vi "Send.vi"(7 "Motors input":refnum<vi>[](array[refnum]), 8 "Error In":errorcluster, 11 "VISA resource name":refnum<visa-resource-name>) -> (0 "Error Out":errorcluster, 3 "VISA resource name out":refnum<visa-resource-name>)   [LabVIEW 2013]
panel:
  out "return count":u32
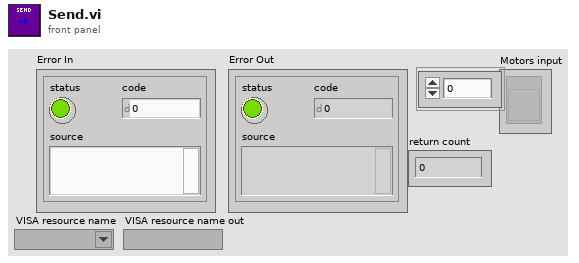
[diagram p1: front panel]
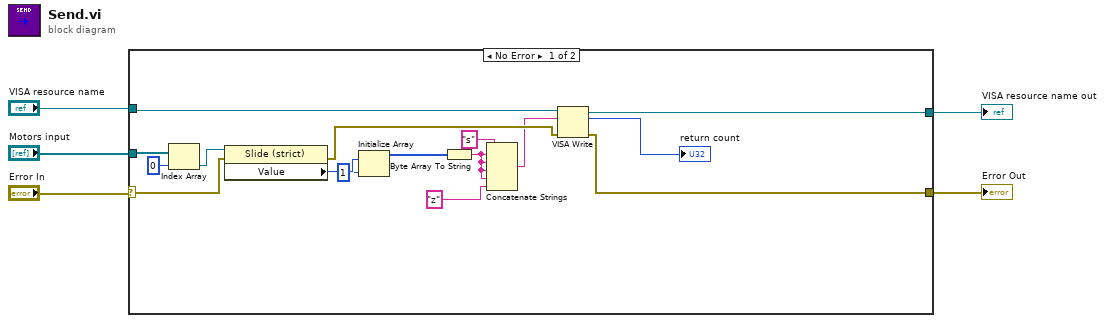
[diagram p0: block diagram]
diagram:
  n1 = case shown="No Error" "Error In" {
    selector: "Error In" -> [w15 w23]
    tunnel: [w11 w23] -> w4
    tunnel: "VISA resource name" -> [w13 w22]
    tunnel: "Motors input" -> [w21 _]
    tunnel: [w14 w22] -> w1
    frame No Error {
      n2 = Index Array(array=w21, index=0) -> (element=w19:refnum<vi>)
      n3 = property class="Slide (strict)"(reference=w19, error in=w15) -> (error out=w12:errorcluster, "Value"=w18:u8)  [unwired: 1 out]
      n4 = Initialize Array(w18, 1 ("dimension size")) -> (w16:u8[])
      n5 = Byte Array To String(unsigned byte array=w16) -> (string=w7:string)
      n6 = Concatenate Strings("s" ("string"), w7, w7, w7, w7, "z" ("string")) -> (w9:string)
      n7 = VISA Write(VISA resource name=w13, write buffer=w9, error in (no error)=w12) -> (VISA resource name out=w14:refnum<visa-resource-name>, return count=→"return count":u32, error out=w11:errorcluster)
    }
    frame Error {
    }
  }
  "Error Out" <- w4
  "VISA resource name out" <- w1
